vi "UpdateCVT[Init].vi"(8 "error in (no error)":errorcluster, 11 "GenericCamera in":refnum<class "GenericCamera.lvclass">) -> (0 "error out":errorcluster, 3 "GenericCamera out":refnum<class "GenericCamera.lvclass">)   [LabVIEW 2013, in "GenericCamera.lvclass"]
uses:
  GenericCamera.lvclass
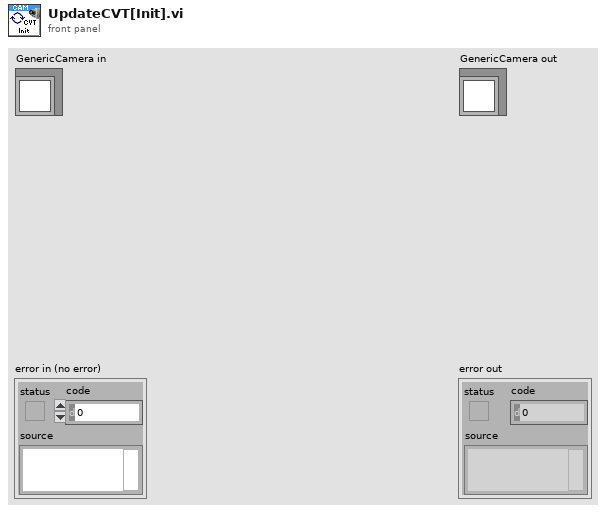
[diagram p1: front panel]
types:
  T1 = cluster{"Value":dbl, "Min":dbl, "Max":dbl, "StepSize":dbl, "Tolerance":dbl, "valueactual":dbl}
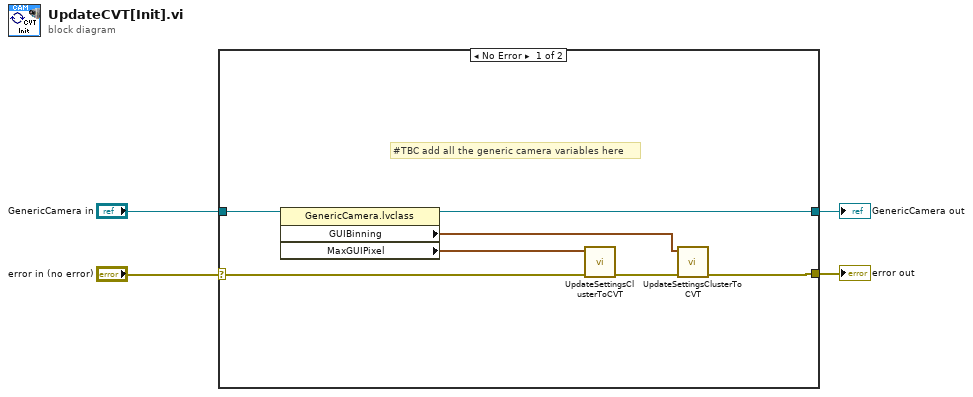
[diagram p0: block diagram]
diagram:
  n1 = case shown="No Error" "error in (no error)" {
    selector: "error in (no error)" -> [w11 w13]
    tunnel: [w7 w13] -> w3
    tunnel: [w5 w12] -> w1
    tunnel: "GenericCamera in" -> [w6 w12]
    frame No Error {
      # "#TBC add all the generic camera variables here"
      n2 = property class="GenericCamera.lvclass"(reference=w6) -> (reference out=w5:refnum<class "GenericCamera.lvclass">, "GUIBinning"=w8:T1, "MaxGUIPixel"=w10:T1)  [unwired: 1 in, 1 out]
      n3 = call "UpdateSettingsClusterToCVT.vi"("error in (no error)"=w11, "variant"=w10) -> ("error out"=w9:errorcluster)  [unwired: 9 in]
      n4 = call "UpdateSettingsClusterToCVT.vi"("error in (no error)"=w9, "variant"=w8) -> ("error out"=w7:errorcluster)  [unwired: 9 in]
    }
    frame Error {
    }
  }
  "error out" <- w3
  "GenericCamera out" <- w1
